vi "type convert.vi"(10 "Task Coordinates Actual (cm)":dbl[](array[numeric]), 11 "Task Coordinates Desired (cm)":dbl[](array[numeric])) -> (3 "Task Coordinates for Buffer Plot":T1(array[cluster]))   [LabVIEW 2017]
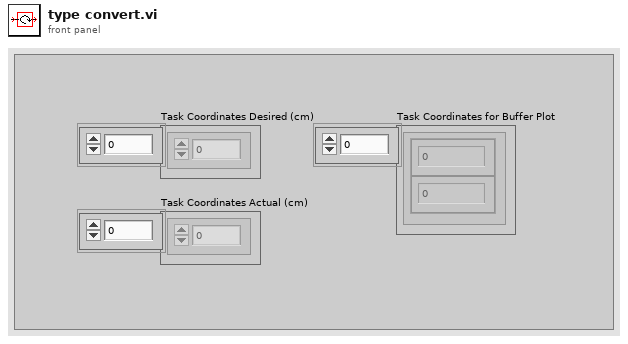
[diagram p1: front panel]
types:
  T1 = cluster{"Numeric Control":dbl, "Numeric Control":dbl}[]
  T2 = cluster{"Numeric Control":dbl, "Numeric Control":dbl}
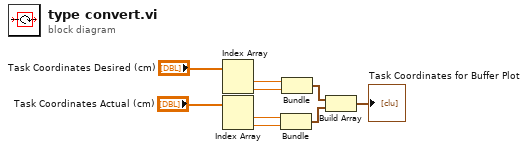
[diagram p0: block diagram]
diagram:
  n1 = Index Array(array="Task Coordinates Desired (cm)") -> (element #1=w3:dbl, element #2=w4:dbl)  [unwired: 2 in]
  n2 = Index Array ("Index Array 2")(array="Task Coordinates Actual (cm)") -> (element #1=w5:dbl, element #2=w6:dbl)  [unwired: 2 in]
  n3 = Bundle ("Bundle 2")("Numeric Control"=w5, "Numeric Control"=w6) -> (w8:T2)  [unwired: 1 in]
  n4 = Bundle("Numeric Control"=w3, "Numeric Control"=w4) -> (w7:T2)  [unwired: 1 in]
  n5 = Build Array ("Build Array 3")(w7, w8) -> (→"Task Coordinates for Buffer Plot":T1)
